vi "EventLogRef Global.vi"() -> ()   [LabVIEW 2019, in "EventLog.lvlib" / "EventLog.lvclass"]
uses:
  EventLog.lvclass
  <vilib>/ActorFramework/Message Enqueuer/Message Enqueuer.lvclass
panel:
  in  "EventLog REF":refnum<class "Message Enqueuer.lvclass">
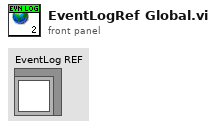
[diagram p1: front panel]
diagram:
